vi "Multirate IIR Filter.vi"() -> ()   [LabVIEW 2023]
doc: "This VI illustrates the use of Stream Channels to create a multi-stage multi-rate IIR resampling filter."
uses:
  <extravilib>/ChannelInstances/Stream-dbl/Read With Abort.vi
  <extravilib>/ChannelInstances/Stream-dbl/Write With Abort.vi
  <extravilib>/ChannelInstances/Stream-dbl/EndpointRead.vi
  <extravilib>/ChannelInstances/Stream-dbl/Endpoint.vi
  <extravilib>/ChannelInstances/Stream-dbl/Instantiate.vi
  <extravilib>/ChannelInstances/Stream-dbl/)Channel.vi
  <resource>/ChannelSupport/_ChannelSupport/WaitIfNeeded.vi
  <extravilib>/ChannelInstances/Stream-dbl.lvlib
panel:
  in  "gain":dbl(slide)=1.0 scale=0.0..2.0
  in  "Stop":bool
  in  "frequency":dbl(knob)=5.0 scale=0.0..10.0 scale format="%.1f"
  out "Output Signal":dbl(graph)
  out "Input Signal":dbl(graph)
  # "Overview: Demonstrates the use of the Stream Channel in making a multi-stage multi-rate IIR filter for resampling an audio waveform.\n\nInstructions:\nRun the VI.  Observe the input data.  Observe the output data to be the same as the input but sampled at half the rate.  Adjust gain and frequency to vary the signal."
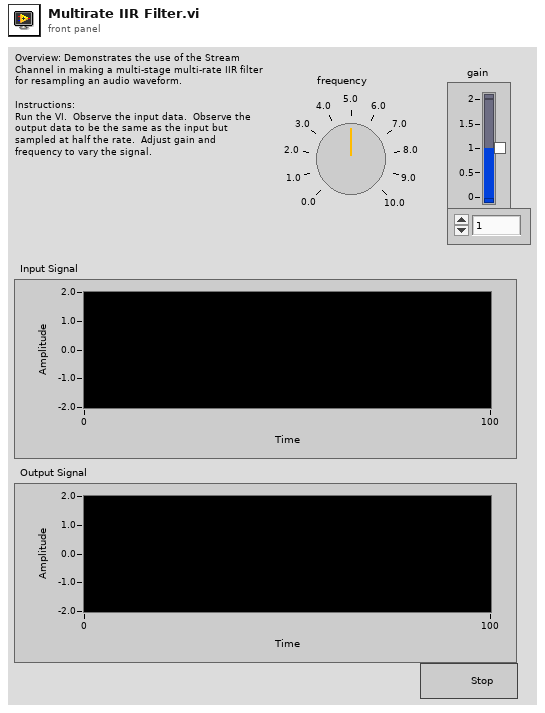
[diagram p1: front panel]
types:
  T1 = typedef "Stream-dbl.lvlib/)Channel.ctl" = refnum<queue>
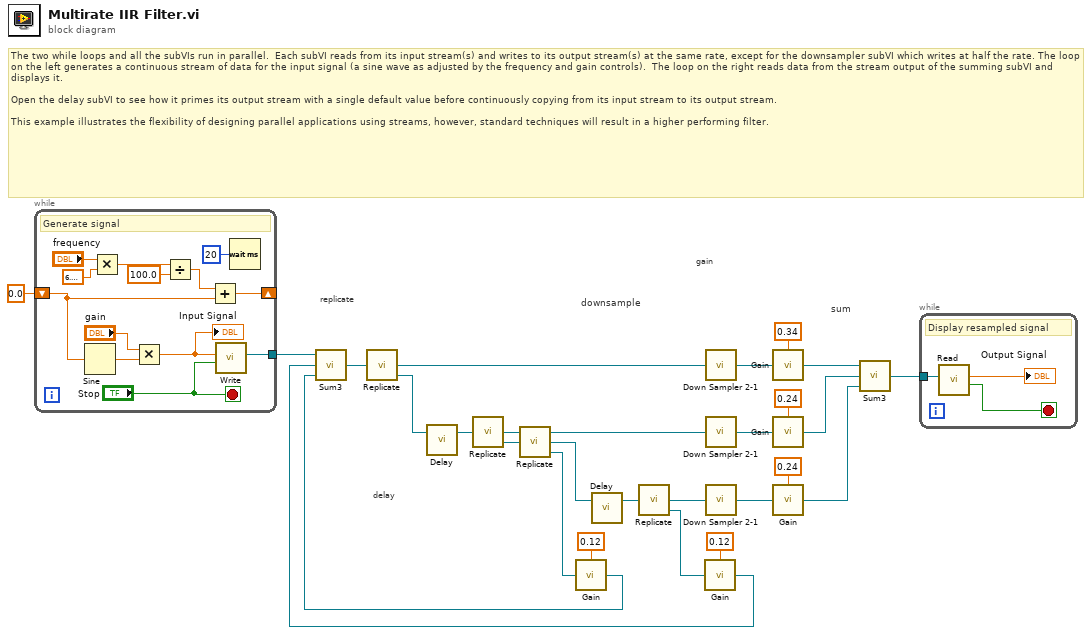
[diagram p0: block diagram]
diagram:
  # "gain"
  # "sum"
  # "replicate"
  # "delay"
  # "downsample"
  # "The two while loops and all the subVIs run in parallel.  Each subVI reads from its input stream(s) and writes to its output stream(s) at the same rate, except for the downsampler subVI which writes at half the rate. The loop on the left generates a continuous stream of data for the input signal (a sine wave as adjusted by the frequency and gain controls).  The loop on the right reads data from the stream output of the summing subVI and displays it.\n\nOpen the delay subVI to see how it primes its output stream with a single default value before continuously copying from its input stream to its output stream.\n\nThis example illustrates the flexibility of designing parallel applications using streams, however, standard techniques will result in a higher performing filter."
  n1 = while {
    shift-right: [w38] -> _
    shift-left: 0.0 -> [w39]
    tunnel: [w29] -> w19
    stop <- "Stop" stop-if-true
    # "Generate signal"
    n2 = Sine(x=w39) -> (sin(x)=w32:dbl)
    n3 = Multiply(x="frequency", y=6.283185307179586) -> (x*y=w35:dbl)
    n4 = Multiply(x="gain", y=w32) -> (x*y=w30:dbl)
    "Input Signal" <- w30
    n5 = Divide(x=w35, y=100.0) -> (x/y=w34:dbl)
    n6 = Add(x=w34, y=w39) -> (x+y=w38:dbl)
    n7 = call <extravilib>:"Write.vi"("last element? (F)"="Stop", "element"=w30) -> ("channel"=w29:T1)  [unwired: 7 in, 2 out]
    n8 = Wait (ms)(milliseconds to wait=u32 20 ("millisecond multiple")) -> ()  [unwired: 1 out]
  }
  n9 = call "Sum3.vi"("stream 3"=w18, "stream 2"=w17, "stream 1"=w19) -> ("stream out"=w11:T1)  [unwired: 1 in]
  n10 = call <extravilib>:"Replicate.vi"("stream"=w11) -> ("stream copy 1"=w10:T1, "stream copy 2"=w9:T1)  [unwired: 7 in]
  n11 = call "Delay.vi"("stream in"=w9) -> ("stream out"=w5:T1)  [unwired: 1 in]
  n12 = call <extravilib>:"Replicate.vi"("stream"=w5) -> ("stream copy 1"=w4:T1, "stream copy 2"=w3:T1)  [unwired: 7 in]
  n13 = call <extravilib>:"Replicate.vi"("stream"=w3) -> ("stream copy 1"=w2:T1, "stream copy 2"=w1:T1)  [unwired: 7 in]
  n14 = call "Gain.vi"("stream in"=w1, "gain"=0.12) -> ("stream out"=w18:T1)
  n15 = call "Delay.vi"("stream in"=w2) -> ("stream out"=w8:T1)  [unwired: 1 in]
  n16 = call <extravilib>:"Replicate.vi"("stream"=w8) -> ("stream copy 1"=w7:T1, "stream copy 2"=w6:T1)  [unwired: 7 in]
  n17 = call "Gain.vi"("stream in"=w6, "gain"=0.12) -> ("stream out"=w17:T1)
  n18 = call "Down Sampler 2-1.vi"("stream in"=w10) -> ("stream out"=w12:T1)
  n19 = call "Down Sampler 2-1.vi"("stream in"=w4) -> ("stream out"=w23:T1)
  n20 = call "Down Sampler 2-1.vi"("stream in"=w7) -> ("stream out"=w22:T1)
  n21 = call "Gain.vi"("stream in"=w12, "gain"=0.34) -> ("stream out"=w16:T1)
  n22 = call "Gain.vi"("stream in"=w23, "gain"=0.24) -> ("stream out"=w14:T1)
  n23 = call "Gain.vi"("stream in"=w22, "gain"=0.24) -> ("stream out"=w13:T1)
  n24 = call "Sum3.vi"("stream 3"=w13, "stream 2"=w14, "stream 1"=w16) -> ("stream out"=w15:T1)  [unwired: 1 in]
  n25 = while {
    tunnel: w15 -> [w43]
    stop <- w41 stop-if-true
    # "Display resampled signal"
    n26 = call <extravilib>:"Read.vi"("channel"=w43) -> ("last element?"=w41:bool, "element"=→"Output Signal":dbl)  [unwired: 6 in, 3 out]
  }
